vi "Wall_Init.vi"(8 "error in (no error)":errorcluster, 10 "Wall Color":u32(colorbox)=32639) -> (0 "error out":errorcluster, 3 "object out":refnum<class "Wall.lvclass">)   [LabVIEW 2017, in "Wall.lvclass"]
uses:
  Wall.lvclass
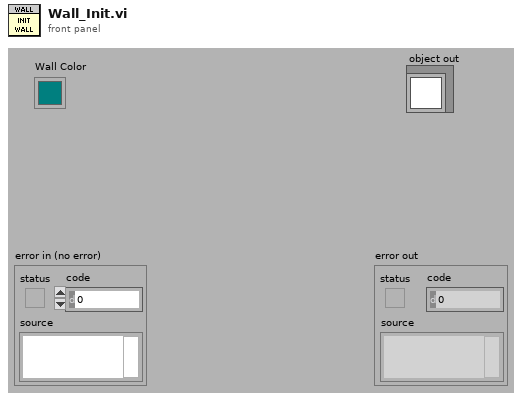
[diagram p1: front panel]
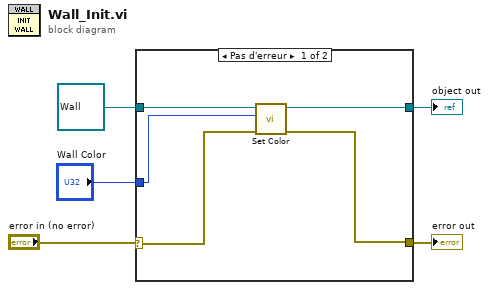
[diagram p0: block diagram]
diagram:
  n1 = case shown="Pas d'erreur" "error in (no error)" {
    selector: "error in (no error)" -> [w8 w11]
    tunnel: [w9 w12] -> w5
    tunnel: refnum<class "Wall.lvclass"> refnum ("object in") -> [w10 w12]
    tunnel: [w7 w11] -> w2
    tunnel: "Wall Color" -> [w6 _]
    frame No Error {
      n2 = call-dynamic "Set Color.vi"("error in (no error)"=w8, "Color"=w6, "object in"=w10) -> ("error out"=w7:errorcluster, "object out"=w9:refnum<class "Wall.lvclass">)  [unwired: 7 in]
    }
    frame Error {
    }
  }
  "object out" <- w5
  "error out" <- w2
